vi "校准信息读取.vi"(8 "Error in":errorcluster caption="Error in (no error)", 11 "Slave ID":u8=1) -> (0 "error out":errorcluster, 3 "校准信息读取":T1 {"校准类型" items=["单点校准"=1, "两点校准"=2, "三点校准"=3]})   [LabVIEW 2016, in "斯坦道原位多参数.lvlib"]
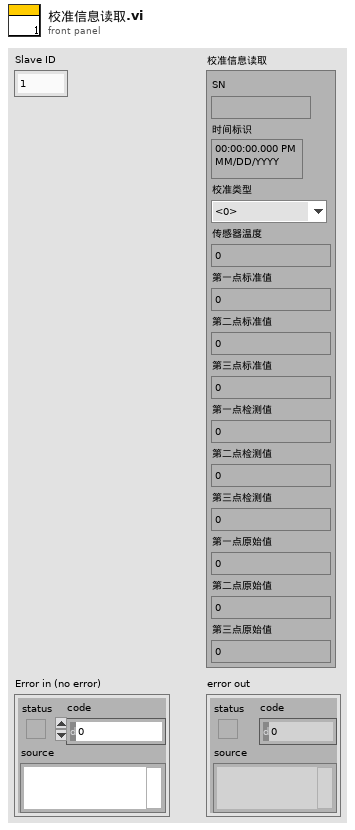
[diagram p1: front panel]
types:
  T1 = cluster{"SN":string, "时间标识":timestamp, "校准类型":u16, "传感器温度":sgl, "第一点标准值":sgl, "第二点标准值":sgl, "第三点标准值":sgl, "第一点检测值":sgl, "第二点检测值":sgl, "第三点检测值":sgl, "第一点原始值":sgl, "第二点原始值":sgl, "第三点原始值":sgl}
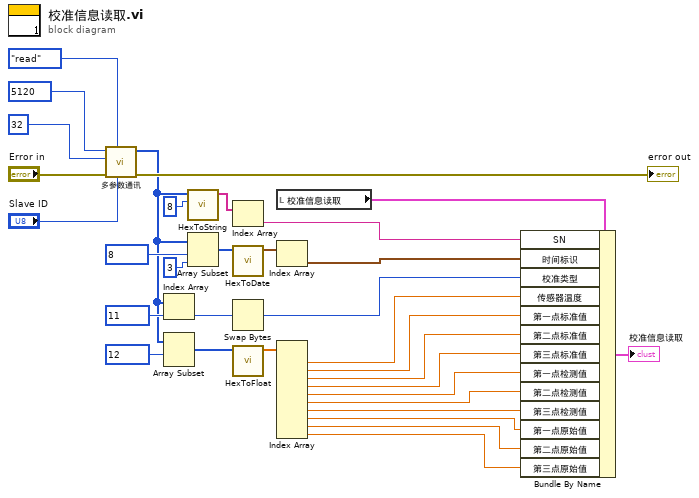
[diagram p0: block diagram]
diagram:
  n1 = call "多参数通讯.vi"("Slave ID"="Slave ID", "STEP"=enum16{"open", "read", "write", "close"}."read", "Error in"="Error in", "quantity"=u16 32, "starting address"=u16 5120) -> ("error out"=→"error out":errorcluster, "Registers"=w22:u16[])  [unwired: 4 in, 1 out]
  n2 = Index Array(array=w22, index=u16 11 ("starting address")) -> (element=w2:u16)
  n3 = Array Subset(array=w22, index=u16 12 ("starting address")) -> (w20:u16[])  [unwired: 1 in]
  n4 = call "HexToString.vi"("字符个数"=8, "数组"=w22) -> ("STRING"=w17:string[])  [unwired: 9 in]
  n5 = Array Subset(array=w22, index=u16 8 ("starting address"), length=3 ("长度")) -> (w24:u16[])
  n6 = Index Array(array=w17) -> (element=w16:string)  [unwired: 1 in]
  n7 = call "HexToDate.vi"("数组"=w24) -> ("DATE"=w15:timestamp[])  [unwired: 10 in]
  n8 = Swap Bytes(anything=w2) -> (byte swapped=w1:u16)
  n9 = call "HexToFloat.vi"("数组"=w20) -> ("FLOAT"=w13:sgl[])  [unwired: 10 in]
  n10 = local read "校准信息读取"() -> (w19:T1)
  n11 = Index Array(array=w15) -> (element=w14:timestamp)  [unwired: 1 in]
  n12 = Index Array(array=w13) -> (element #1=w12:sgl, element #2=w11:sgl, element #3=w10:sgl, element #4=w9:sgl, element #5=w8:sgl, element #6=w7:sgl, element #7=w6:sgl, element #8=w5:sgl, element #9=w4:sgl, element #10=w3:sgl)  [unwired: 10 in]
  n13 = Bundle By Name(cluster=w19, "SN"=w16, "时间标识"=w14, "校准类型"=w1, "传感器温度"=w12, "第一点标准值"=w11, "第二点标准值"=w10, "第三点标准值"=w9, "第一点检测值"=w8, "第二点检测值"=w7, "第三点检测值"=w6, "第一点原始值"=w5, "第二点原始值"=w4, "第三点原始值"=w3) -> (→"校准信息读取":T1)
